vi "Configure Block Notify.vi"(7 "Notify ID (0: Notify 1)":i32(ring) items=["Notify 1", "Notify 2", "Notify 3", "Notify 4", "Notify 5", "Notify 6", "Notify 7", "Notify 8"], 8 "error in (no error)":errorcluster, 10 "Block Number (0)":u32, 11 "VISA resource name":refnum<visa-resource-name>) -> (0 "error out":errorcluster, 3 "VISA resource name out":refnum<visa-resource-name>)   [LabVIEW 2016, in "Keithley DMM6500 DAQ6500 Series.lvlib"]
doc: "Defines a trigger model block that generates a trigger event and immediately continues to the next block."
uses:
  Keithley DMM6500 DAQ6500 Series.lvlib
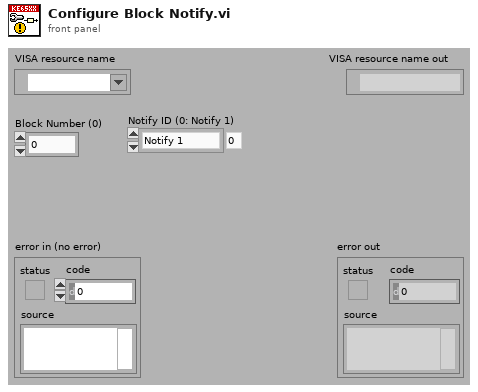
[diagram p1: front panel]
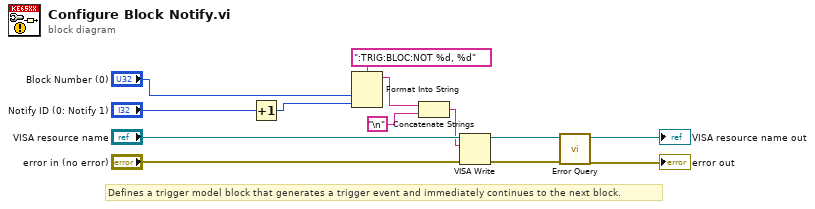
[diagram p0: block diagram]
diagram:
  # "Defines a trigger model block that generates a trigger event and immediately continues to the next block."
  n1 = Increment(x="Notify ID (0: Notify 1)") -> (x+1=w1:i32)
  n2 = Format Into String(format string=":TRIG:BLOC:NOT %d, %d", "Block Number (0)", w1) -> (resulting string=w4:string)  [unwired: 2 in, 1 out]
  n3 = Concatenate Strings(w4, "\n") -> (w5:string)
  n4 = VISA Write(VISA resource name="VISA resource name", write buffer=w5, error in (no error)="error in (no error)") -> (VISA resource name out=w9:refnum<visa-resource-name>, error out=w8:errorcluster)  [unwired: 1 out]
  n5 = call "Error Query.vi"("error in (no error)"=w8, "VISA resource name"=w9) -> ("error out"=→"error out":errorcluster, "VISA resource name out"=→"VISA resource name out":refnum<visa-resource-name>)  [unwired: 6 in, 2 out]
